vi "预处理部分.vi"() -> (0 "error out":errorcluster, 1 "干净语音信号":dbl[](array[numeric]), 2 "s2":dbl, 3 "s1":dbl, 4 "y":dbl[][](array[numeric]))   [LabVIEW 2013]
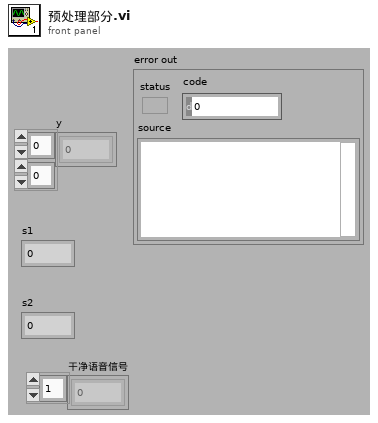
[diagram p1: front panel]
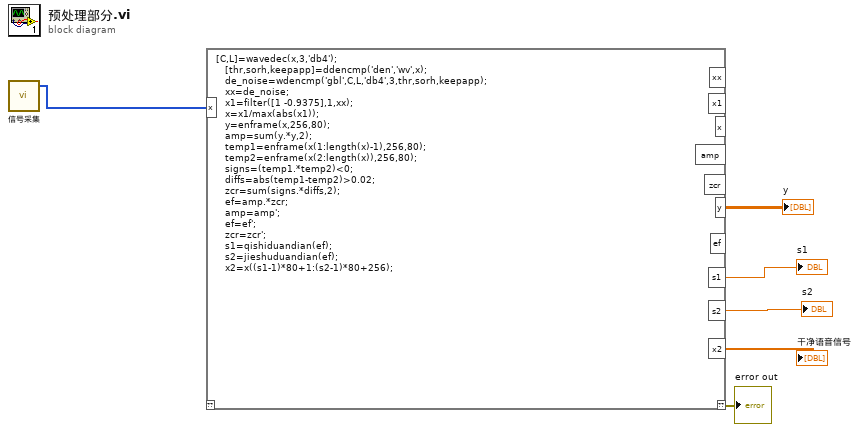
[diagram p0: block diagram]
diagram:
  n1 = call "信号采集.vi"() -> ("波形图"=w1:i16[])  [unwired: 1 in, 1 out]
  n2 = script code="[C,L]=wavedec(x,3,'db4');\n   [thr,sorh,keepapp]=ddencmp('den','wv',x);\n   de_noise=wdencmp('gbl',C,L,'db4',3,thr,sorh,keepapp);\n   xx=de_noise;\n   x1=filter([1 -0.9375],1,xx);\n   x=x1/max(abs(x1));\n   y=enframe(x,256,80);\n   amp=sum(y.*y,2);\n   temp1=enframe(x(1:length(x)-1),256,80);\n   temp2=enframe(x(2:length(x)),256,80);\n   signs=(temp1.*temp2)<0;\n   diffs=abs(temp1-temp2)>0.02;\n   zcr=sum(signs.*diffs,2);\n   ef=amp.*zcr;\n   amp=amp';\n   ef=ef';\n   zcr=zcr';\n   s1=qishiduandian(ef);\n   s2=jieshuduandian(ef);\n   x2=x((s1-1)*80+1:(s2-1)*80+256);"("x"=w1) -> ("??"=→"error out":errorcluster, "y"=→"y":dbl[][], "s1"=→"s1":dbl, "s2"=→"s2":dbl, "x2"=→"干净语音信号":dbl[])  [unwired: 1 in, 6 out]
